vi "SampleGUI.vi"() -> ()   [LabVIEW 2017]
uses:
  <vilib>/LabVIEW Interface for Arduino/Type Defs/Board Type.ctl
  <vilib>/LabVIEW Interface for Arduino/Type Defs/Connection Type.ctl
  <vilib>/LabVIEW Interface for Arduino/Type Defs/Pin Mode.ctl
  <vilib>/LabVIEW Interface for Arduino/LabVIEW Interface for Arduino.lvlib
panel:
  in  "Auto Abort":bool
  out "error out":errorcluster
  in  "stop":bool
  in  "Relief\nPiston":bool
  in  "Fuel":bool
  out "High\nVibration":bool
  out "Max Pressure":bool
  out "Oxidizer\nPressure":bool
  in  "Abort  Sequence":bool
  out "Fuel \nPressure":bool
  in  "Pressurant":bool
  in  "Oxidizer":bool
  in  "Tab Control":enum32{"Burn Display", "Data Log", "Procedures"}(tab)
  out "Peak Thrust":dbl
  out "Total Impulse":dbl
  out "Average Thrust":dbl
  out "Total Samples":dbl
  out "Burn Time":dbl
  out "Load Cell 2":dbl[](graph)
  out "Load Cell 1":dbl[](graph)
  out "Load Cell 4":dbl[](graph)
  out "Load Cell 3":dbl[](graph)
  out "Oxidizer":u8(slide) scale=0.0..100.0
  out "Fuel":u8(slide) scale=0.0..100.0
  out "String":string
  # "Valves"
  # "Warnings"
  # "Abort"
  # "SEB Static Test"
  # "Engine Performance Dashboard"
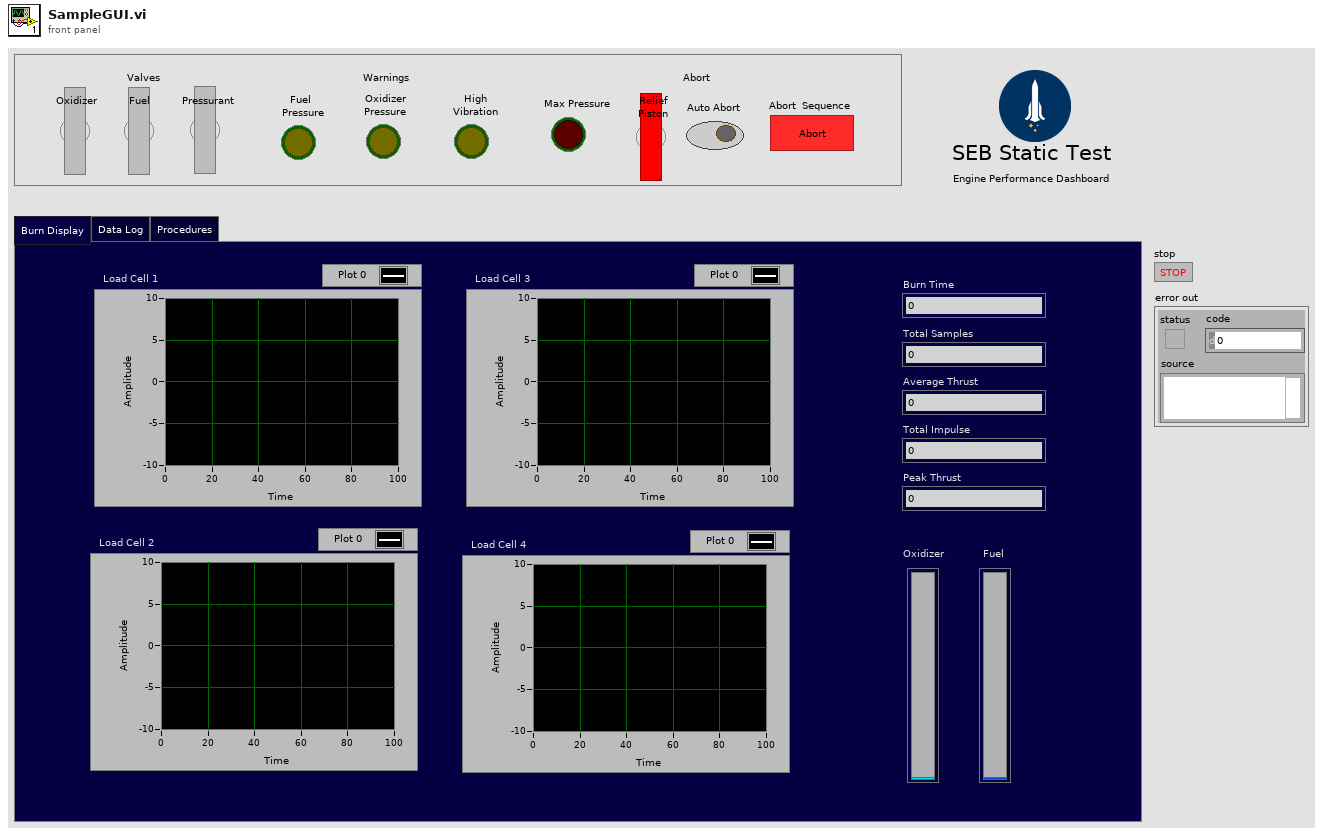
[diagram p1: front panel]
types:
  T1 = typedef "LabVIEW Interface for Arduino.lvlib/Pin Mode.ctl" = enum8{"Input", "Output"}
  T2 = typedef "LabVIEW Interface for Arduino.lvlib/Connection Type.ctl" = enum8{"USB / Serial", "XBEE", "BlueSmirf (Bluetooth)"}
  T3 = typedef "LabVIEW Interface for Arduino.lvlib/Board Type.ctl" = enum16{"Uno", "Dimuelanove w/Atmega 328", "Mega 2560"}
  T4 = typedef "LabVIEW Interface for Arduino.lvlib/Arduino Resource.ctl" = cluster{"VISA resource":refnum<visa-resource-name>, "Board Type":T3, "Connection Type":enum8{"USB / Serial"}, "Bytes Per Packet (15)":u8}
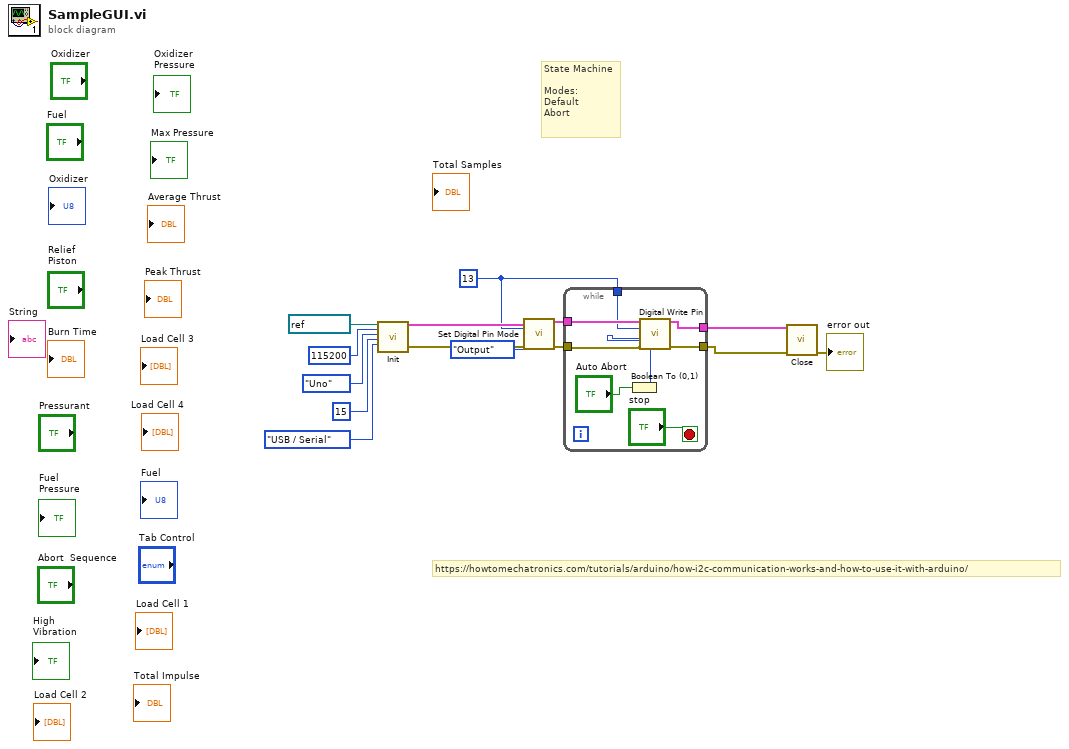
[diagram p0: block diagram]
diagram:
  w4 = u8 13 ("Digital I/O Pin")
  # "https://howtomechatronics.com/tutorials/arduino/how-i2c-communication-works-and-how-to-use-it-with-arduino/"
  # "State Machine\n\nModes:\nDefault\nAbort"
  n1 = call <vilib>:"Init.vi"("VISA resource"=refnum<visa-resource-name> "COM3", "Baud Rate (115200)"=u32 115200, "Board Type (Uno)"=Board_Type."Uno", "Bytes Per Packet (15)"=u32 15, "Connection Type (USB/Serial)"=Connection_Type."USB / Serial") -> ("Arduino Resource"=w9:T4, "error out"=w5:errorcluster)  [unwired: 13 in]
  n2 = call <vilib>:"Set Digital Pin Mode.vi"("Arduino Resource"=w9, "Digital I/O Pin"=w4, "Pin Mode (Input)"=Pin_Mode."Output", "error in"=w5) -> ("Arduino Resource"=w7:T4, "error out"=w6:errorcluster)  [unwired: 10 in]
  n3 = while {
    tunnel: w7 -> [w22]
    tunnel: w6 -> [w20]
    tunnel: w4 -> [w21]
    tunnel: [w19] -> w2
    tunnel: [w17] -> w3
    stop <- "stop" stop-if-true
    n4 = Boolean To (0,1)(Boolean="Auto Abort") -> (0, 1=w15:i16)
    n5 = call <vilib>:"Digital Write Pin.vi"("Arduino Resource"=w22, "Digital I/O Pin (0)"=w21, "Value (0)"=w15, "error in"=w20) -> ("Arduino Resource"=w17:T4, "error out"=w19:errorcluster)  [unwired: 10 in]
  }
  n6 = call <vilib>:"Close.vi"("Arduino Resource"=w3, "error in"=w2) -> ("error out"=→"error out":errorcluster)  [unwired: 13 in]
